vi "Adaptive Filter 3.vi"(4 "Beta":fxp<+/-,32,-16>, 6 "Noise":T3, 8 "Memory":T2, 10 "Filter Size":i32, 11 "Input":fxp<+/-,16,16>) -> (0 "Data":T1 {"BetaProduct" format="%.33g"; "WeightSum" format="%.20g"}, 3 "Error Out":fxp<+/-,16,16> format="%.16g")   [LabVIEW 2016]
uses:
  MemoryBlocks.ctl
  <vilib>/Platform/TimedLoop/XDataNode/timing_clust.ctl
  <vilib>/Platform/TimedLoop/XDataNode/nitl_modes.ctl
  <vilib>/Platform/TimedLoop/XDataNode/wakeup.ctl
  <vilib>/rvi/Emulation/niFpgaSctlEmulationGetInTimedLoop.vi
  <vilib>/rvi/Emulation/niFpgaEmulationReportErrorSimple.vi
  <vilib>/rvi/Emulation/niFpgaGetClockAttributes.vi
  <vilib>/rvi/Emulation/niFpgaCriticalErrorInLSC.vi
  <vilib>/rvi/DataTransferAndStorage/Container/Common/niFpgaContainerExecOnDevCompGetState.vi
  <vilib>/rvi/Emulation/niFpgaEmulationIsFPGAContextNoSignature.vi
  <vilib>/rvi/DataTransferAndStorage/Container/Common/niFpgaContainerGetUniqueNameForEmu.vi
  <vilib>/rvi/Emulation/niFpgaProcessEmulError.vi
  <vilib>/rvi/errors/nirviReportUnexpectedCaseInternalError (U32).vi
  <vilib>/rvi/Memory/Memory_Emulation/niFpgaMemoryEmulationCacheClearOnFirstRun.vi
  <vilib>/rvi/Memory/Memory_Emulation/nirvimemoryEmulationManagerCache_MakeExclusive.vi
  <vilib>/rvi/Memory/Memory_Emulation/niFpgaMemoryEmulationValidateCache.vi
  <vilib>/rvi/Memory/Memory_Emulation/nirvimemoryEmulationManagerCache_InsertValue.vi
  <vilib>/Utility/error.llb/Clear Errors.vi
  <vilib>/rvi/Memory/Memory_Emulation/nirvimemoryEmulationManagerCache_ReleaseExclusive.vi
  <vilib>/rvi/Memory/Memory_Emulation/nirvimemoryEmulationManagerCache_GetValue.vi
  <vilib>/rvi/Memory/Memory_Emulation/nirvimemoryEmulationManagerCache_SetValue.vi
  <vilib>/rvi/Emulation/niFpgaSctlEmulationResourceMgr.vi
  <vilib>/Platform/TimedLoop/XDataNode/XDataNode.xnode
  <vilib>/rvi/DataTransferAndStorage/Container/XNode/niFpgaContainer.xnode
  <vilib>/rvi/Memory/Memory_Emulation/niFpgaMemoryEmulationRefIn.vi
  <vilib>/Platform/TimedLoop/XDataNode/XDNodeRunTimeDep.lvlib
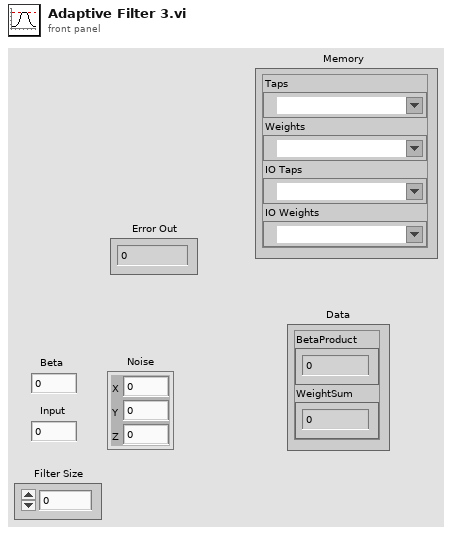
[diagram p1: front panel]
types:
  T1 = cluster{"BetaProduct":fxp<+/-,32,-1>, "WeightSum":fxp<+/-,33,19>}
  T2 = typedef "MemoryBlocks.ctl" = cluster{"Taps":refnum<k21>, "Weights":refnum<k21>, "IO Weights":refnum<k21>, "IO Taps":refnum<k21>}
  T3 = cluster{"X":fxp<+/-,16,16>, "Y":fxp<+/-,16,16>, "Z":fxp<+/-,16,16>}
  T4 = typedef "XDNodeRunTimeDep.lvlib/timing_clust.ctl" = cluster{"Expected End [f-1]":u64, "Actual End [f-1]":u64, "Finished Late? [f-1]":bool, "Expected End [i-1]":u64, "Actual End [i-1]":u64, "Finished Late? [i-1]":bool, "Expected Start [i]":u64, "Actual Start [i]":u64, "Expected Start [f]":u64, "Actual Start [f]":u64, "Source Name":string, "Structure Name":string, "Period":i64, "Deadline":i64, "Offset":i64, "Start":i64, "Priority":i32, "Timeout":i32, "Mode":T5, "Wakeup Reason":T6, "Error":errorcluster, "Source Type":string, "Secondary Source Type":string, "Global End Time":u64, "Global Start Time":u64, "Frame Duration":u64, "Iteration Duration":u64, "Assigned CPU":i32, "I/O Scan Engine Mode":u32}
  T5 = typedef "XDNodeRunTimeDep.lvlib/nitl_modes.ctl" = enum32{"No Change", "Process missed periods, maintain original phase", "Discard missed periods, maintain original phase", "Process missed periods, ignore original phase", "Discard missed periods, ignore original phase"}
  T6 = typedef "XDNodeRunTimeDep.lvlib/wakeup.ctl" = enum32{"Normal", "Aborted", "Asynchronous wakeup", "Timing source error", "Timed loop error", "Timeout"}
  T7 = cluster{"fixed-point type":fxp<+/-,32,-1>, "x+y":fxp<+/-,33,19>}
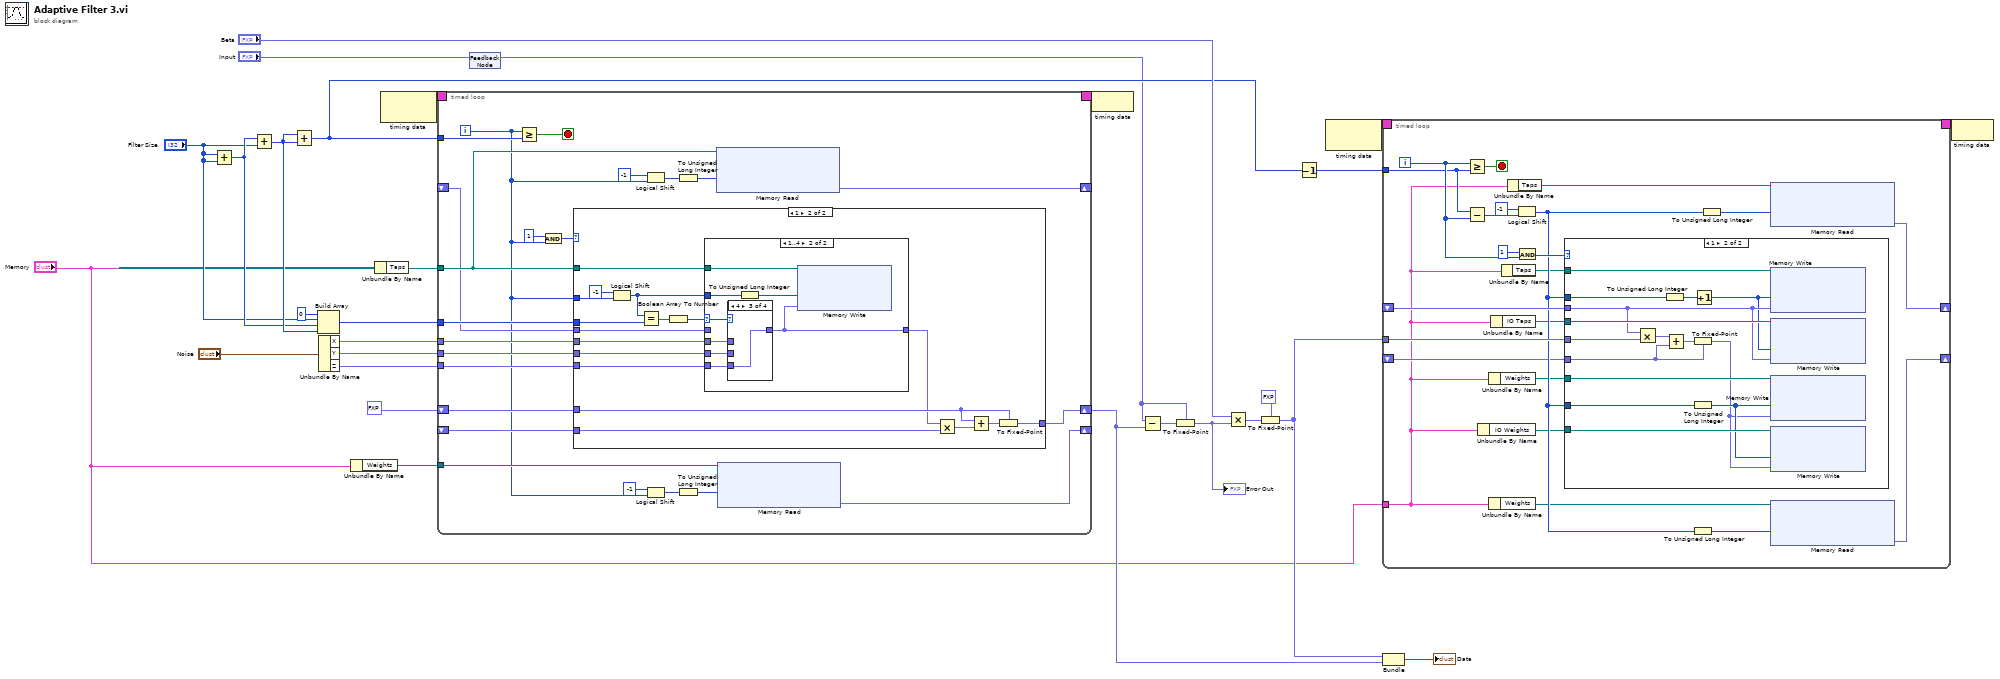
[diagram p0: block diagram]
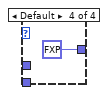
[diagram p7: hidden frame]
diagram:
  n1 = Add(x="Filter Size", y="Filter Size") -> (x+y=w14:i32)
  n2 = Add(x=w14, y="Filter Size") -> (x+y=w15:i32)
  n3 = Add(x=w15, y=w15) -> (x+y=w10:i32)
  n4 = Build Array(0 ("element"), "Filter Size", w14, w15) -> (w16:i32[])
  n5 = Unbundle By Name("Noise") -> ("X"=w28:fxp<+/-,16,16>, "Y"=w27:fxp<+/-,16,16>, "Z"=w26:fxp<+/-,16,16>)
  n6 = Unbundle By Name("Memory") -> ("Weights"=w5:refnum<k21>)
  n7 = Unbundle By Name("Memory") -> ("Taps"=w6:refnum<k21>)
  n8 = node-c288() -> (w24:T4)  [unwired: 1 in]
  n9 = timed-loop {
    tunnel: w6 -> [w41]
    tunnel: w28 -> [w47]
    tunnel: w27 -> [w48]
    tunnel: w26 -> [w49]
    tunnel: w5 -> [w44]
    shift-right: [w51] -> w3
    shift-left: fxp<+/-,33,19> 0.0 ("x+y") -> [w52]
    timing: w24 -> [_]
    timing-out: [_] -> w23
    tunnel: w10 -> [w50]
    shift-right: [w46] -> _
    shift-left: _ -> [w45]
    tunnel: w16 -> [w42]
    shift-right: [w40] -> _
    shift-left: _ -> [w39]
    i -> [w32]
    stop <- w43 stop-if-true
    n10 = Greater Or Equal?(x=w32, y=w50) -> (x >= y?=w43:bool)
    n11 = And(x=1 ("y"), y=w32) -> (x .and. y?=w33:i32)
    n12 = case shown="1" w33 {
      tunnel: w52 -> [w53 w70]
      tunnel: [w53 w69] -> w51
      tunnel: w49 -> [_ w68]
      tunnel: w48 -> [_ w67]
      tunnel: w47 -> [_ w66]
      tunnel: w45 -> [_ w63]
      tunnel: w42 -> [_ w62]
      tunnel: w41 -> [_ w55]
      tunnel: w39 -> [_ w59]
      tunnel: w32 -> [_ w57]
      frame 0, Default {
      }
      frame 1 {
        n13 = Logical Shift(y=i16 -1, x=w57) -> (x << y=w54:i32)
        n14 = Equal?(x=w54, y=w62) -> (x = y?=w61:bool[])
        n15 = Boolean Array To Number(Boolean array=w61) -> (number=w60:u8)
        n16 = case shown="1..4" w60 {
          selector: w60 -> [_ w75]
          tunnel: w55 -> [_ w79]
          tunnel: w68 -> [_ w78]
          tunnel: w67 -> [_ w77]
          tunnel: w66 -> [_ w76]
          tunnel: w59 -> [w71 _]
          tunnel: [w71 w74] -> w56
          tunnel: w54 -> [_ w73]
          frame Default {
          }
          frame 1..4 {
            n17 = case shown="4" w75 {
              tunnel: w76 -> [w80 _ _ _]
              tunnel: w77 -> [_ w81 _ _]
              tunnel: w78 -> [_ _ w82 _]
              tunnel: [w80 w81 w82 fxp<+/-,16,16> 0.0 ("Z")] -> w74
              frame 1 {
              }
              frame 2 {
              }
              frame 4 {
              }
              frame Default {
              }
            }
            n18 = To Unsigned Long Integer(number=w73) -> (unsigned 32bit integer=w72:u32)
            n19 = xnode ("Memory Write")("Address"=w72, "Data"=w74, "Memory In"=w79) -> ()  [unwired: 1 out]
          }
        }
        n20 = Multiply(x=w56, y=w63) -> (x*y=w65:fxp<+/-,40,24>)
        n21 = Add(x=w70, y=w65) -> (x+y=w64:fxp<+/-,40,24>)
        n22 = To Fixed-Point(fixed-point type=w70, number=w64) -> (fixed-point=w69:fxp<+/-,33,19>)
      }
    }
    n23 = Logical Shift(y=i16 -1, x=w32) -> (x << y=w37:i32)
    n24 = Logical Shift(y=i16 -1, x=w32) -> (x << y=w35:i32)
    n25 = To Unsigned Long Integer(number=w37) -> (unsigned 32bit integer=w31:u32)
    n26 = To Unsigned Long Integer(number=w35) -> (unsigned 32bit integer=w30:u32)
    n27 = xnode ("Memory Read")("Address"=w31, "Memory In"=w41) -> ("Data"=w40:fxp<+/-,16,16>)  [unwired: 1 out]
    n28 = xnode ("Memory Read")("Address"=w30, "Memory In"=w44) -> ("Data"=w46:fxp<+/-,24,8>)  [unwired: 1 out]
  }
  n29 = feedback-in #1("Input") -> ()
  n30 = feedback #1() -> (w7:fxp<+/-,16,16>)  [unwired: 1 in]
  n31 = node-c288(w23) -> ()
  n32 = Subtract(x=w7, y=w3) -> (x-y=w25:fxp<+/-,34,20>)
  n33 = To Fixed-Point(fixed-point type=w7, number=w25) -> (fixed-point=w11:fxp<+/-,16,16>)
  "Error Out" <- w11
  n34 = Multiply(x="Beta", y=w11) -> (x*y=w8:fxp<+/-,48,0>)
  n35 = To Fixed-Point(fixed-point type=fxp<+/-,32,-1> 0.0, number=w8) -> (fixed-point=w4:fxp<+/-,32,-1>)
  n36 = Decrement(x=w10) -> (x-1=w9:i32)
  n37 = node-c288() -> (w22:T4)  [unwired: 1 in]
  n38 = timed-loop {
    tunnel: w4 -> [w107]
    timing: w22 -> [_]
    timing-out: [_] -> w21
    tunnel: w9 -> [w98]
    shift-right: [w87] -> _
    shift-left: _ -> [w103]
    shift-right: [w92] -> _
    shift-left: _ -> [w94]
    tunnel: "Memory" -> [w86]
    i -> [w100]
    stop <- w106 stop-if-true
    n39 = Greater Or Equal?(x=w100, y=w98) -> (x >= y?=w106:bool)
    n40 = Subtract(x=w98, y=w100) -> (x-y=w104:i32)
    n41 = Unbundle By Name(w86) -> ("IO Weights"=w96:refnum<k21>)
    n42 = Unbundle By Name(w86) -> ("Weights"=w91:refnum<k21>)
    n43 = Unbundle By Name(w86) -> ("Weights"=w95:refnum<k21>)
    n44 = Unbundle By Name(w86) -> ("IO Taps"=w97:refnum<k21>)
    n45 = Unbundle By Name(w86) -> ("Taps"=w90:refnum<k21>)
    n46 = Unbundle By Name(w86) -> ("Taps"=w89:refnum<k21>)
    n47 = Logical Shift(y=i16 -1, x=w104) -> (x << y=w99:i32)
    n48 = And(x=1, y=w100) -> (x .and. y?=w101:i32)
    n49 = case shown="1" w101 {
      tunnel: w107 -> [_ w122]
      tunnel: w91 -> [_ w121]
      tunnel: w90 -> [_ w120]
      tunnel: w94 -> [_ w118]
      tunnel: w103 -> [_ w111]
      tunnel: w99 -> [_ w117]
      tunnel: w99 -> [_ w115]
      tunnel: w97 -> [_ w113]
      tunnel: w96 -> [_ w112]
      frame 0, Default {
      }
      frame 1 {
        n50 = Multiply(x=w111, y=w122) -> (x*y=w114:fxp<+/-,48,15>)
        n51 = To Unsigned Long Integer(number=w117) -> (unsigned 32bit integer=w116:u32)
        n52 = Add(x=w114, y=w118) -> (x+y=w119:fxp<+/-,48,15>)
        n53 = To Fixed-Point(fixed-point type=w118, number=w119) -> (fixed-point=w108:fxp<+/-,24,8>)
        n54 = To Unsigned Long Integer(number=w115) -> (unsigned 32bit integer=w109:u32)
        n55 = Increment(x=w116) -> (x+1=w110:u32)
        n56 = xnode ("Memory Write")("Address"=w110, "Data"=w111, "Memory In"=w120) -> ()  [unwired: 1 out]
        n57 = xnode ("Memory Write")("Address"=w110, "Data"=w111, "Memory In"=w113) -> ()  [unwired: 1 out]
        n58 = xnode ("Memory Write")("Address"=w109, "Data"=w108, "Memory In"=w121) -> ()  [unwired: 1 out]
        n59 = xnode ("Memory Write")("Address"=w109, "Data"=w108, "Memory In"=w112) -> ()  [unwired: 1 out]
      }
    }
    n60 = To Unsigned Long Integer(number=w99) -> (unsigned 32bit integer=w93:u32)
    n61 = To Unsigned Long Integer(number=w99) -> (unsigned 32bit integer=w88:u32)
    n62 = xnode ("Memory Read")("Address"=w88, "Memory In"=w89) -> ("Data"=w87:fxp<+/-,16,16>)  [unwired: 1 out]
    n63 = xnode ("Memory Read")("Address"=w93, "Memory In"=w95) -> ("Data"=w92:fxp<+/-,24,8>)  [unwired: 1 out]
  }
  n64 = Bundle("fixed-point type"=w4, "x+y"=w3) -> (→"Data":T7)  [unwired: 1 in]
  n65 = node-c288(w21) -> ()
